vi "run vis.vi"(8 "error in (no error)":errorcluster, 11 "home path":path) -> (0 "run vis Error":errorcluster[][](array[cluster]), 2 "Panel VI names":string[](array[string]), 3 "Panel VI paths":path[](array[path]))   [LabVIEW 2016, in "main.lvlib"]
doc: "run vis.VI initializes the Control environment by opening the necessary VIs \nfor operations. \n\nBeamline section controls (main control lower panel): Both sample changers and injectors, low energy end, high energy end, transmission line, and the R30 and R45 beamlines\n\nTools (main control upper panel): monitors for terminal voltage, beam current along with BPM, foil, and other various controls.\n\nTop-level VIs (full VI's opened \"outside\" of main control): sample changer monitor/controller, vacuum readbacks, beam current monitor, cRIO monitor"
uses:
  main.lvlib
panel:
  out "Top Level open errors":errorcluster[](array[cluster])
  out "Top Level run errors":errorcluster[](array[cluster])
  out "Panel VI run errors":errorcluster[](array[cluster])
  out "Top Level paths":path[](array[path])
  out "Numeric 2":i32
  out "Numeric":i32
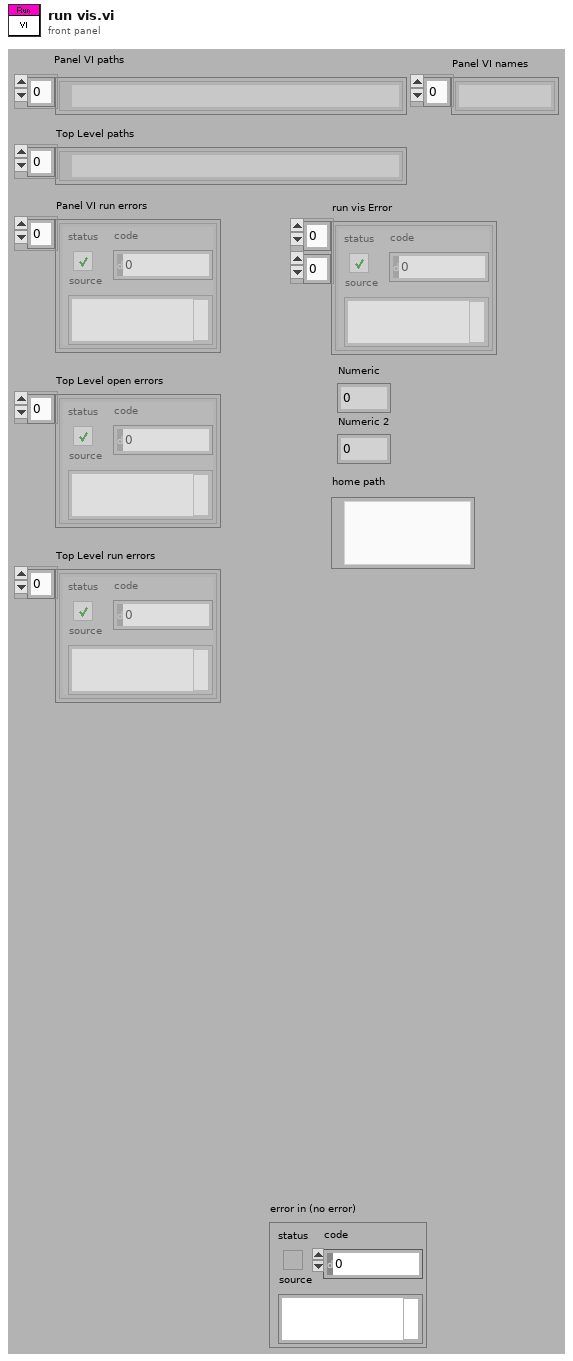
[diagram p1: front panel]
types:
  T1 = enum32{"Invalid", "Standard", "Closed", "Hidden", "Minimized", "Maximized"}
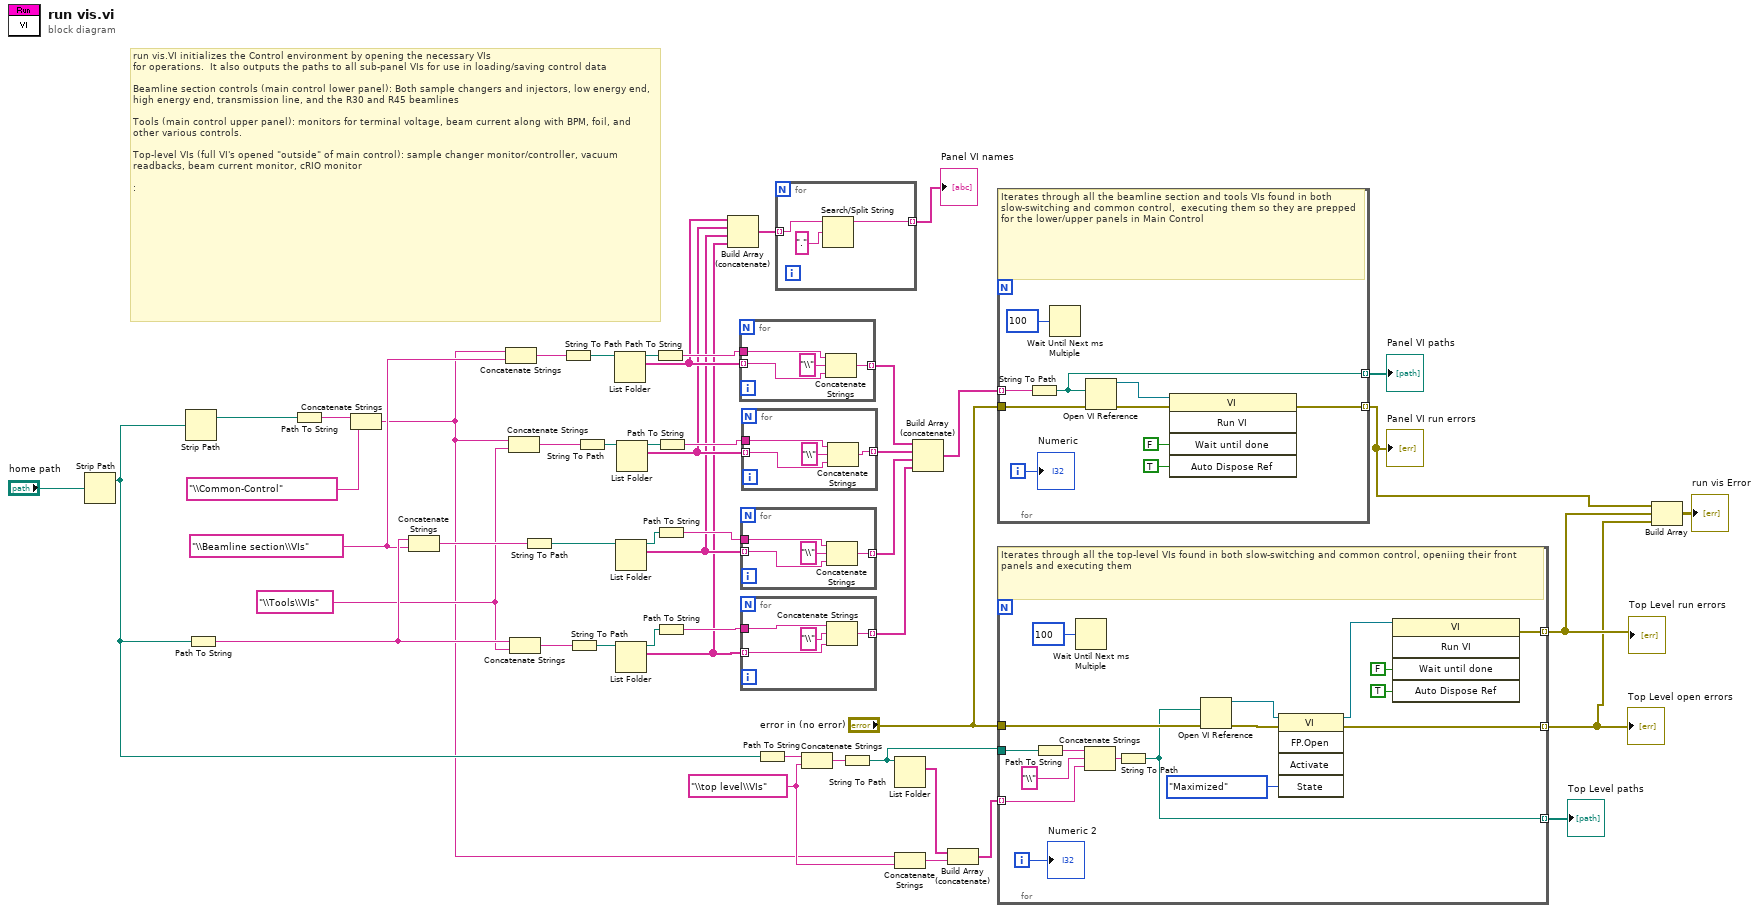
[diagram p0: block diagram]
diagram:
  w15 = "\\top level\\VIs" ("string")
  w27 = "\\Tools\\VIs" ("string")
  w28 = "\\Beamline section\\VIs" ("string")
  # "run vis.VI initializes the Control environment by opening the necessary VIs \nfor operations.  It also outputs the paths to all sub-panel VIs for use in loading/saving control data \n\nBeamline section controls (main control lower panel): Both sample changers and injectors, low energy end, high energy end, transmission line, and the R30 and R45 beamlines\n\nTools (main control upper panel): monitors for terminal voltage, beam current along with BPM, foil, and other various controls.\n\nTop-level VIs (full VI's opened \"outside\" of main control): sample changer monitor/controller, vacuum readbacks, beam current monitor, cRIO monitor\n\n:"
  n1 = Strip Path(path="home path") -> (stripped path=w31:path)  [unwired: 1 out]
  n2 = Strip Path(path=w31) -> (stripped path=w30:path)  [unwired: 1 out]
  n3 = Path To String(path=w31) -> (string=w46:string)
  n4 = Path To String(path=w30) -> (string=w29:string)
  n5 = Concatenate Strings(w29, "\\Common-Control" ("string")) -> (w14:string)
  n6 = Concatenate Strings(w46, w28) -> (w48:string)
  n7 = Concatenate Strings(w14, w28) -> (w24:string)
  n8 = Concatenate Strings(w14, w27) -> (w19:string)
  n9 = Concatenate Strings(w46, w27) -> (w45:string)
  n10 = String To Path(string=w48) -> (path=w47:path)
  n11 = String To Path(string=w24) -> (path=w23:path)
  n12 = String To Path(string=w45) -> (path=w44:path)
  n13 = String To Path(string=w19) -> (path=w20:path)
  n14 = List Folder(path=w23) -> (path out=w25:path, filenames=w6:string[])  [unwired: 3 in, 2 out]
  n15 = List Folder(path=w47) -> (path out=w34:path, filenames=w4:string[])  [unwired: 3 in, 2 out]
  n16 = List Folder(path=w44) -> (path out=w37:path, filenames=w3:string[])  [unwired: 3 in, 2 out]
  n17 = List Folder(path=w20) -> (path out=w21:path, filenames=w5:string[])  [unwired: 3 in, 2 out]
  n18 = Path To String(path=w25) -> (string=w26:string)
  n19 = Path To String(path=w34) -> (string=w35:string)
  n20 = Path To String(path=w37) -> (string=w36:string)
  n21 = Path To String(path=w21) -> (string=w22:string)
  n22 = Build Array (concatenate)(w6, w5, w4, w3) -> (w2:string[])
  n23 = for {
    tunnel: w26 -> [w54]
    tunnel: w6 -> [w52] mode=indexing
    tunnel: [w51] -> w17 mode=indexing
    n24 = Concatenate Strings(w54, "\\" ("string"), w52) -> (w51:string)
  }
  n25 = for {
    tunnel: w35 -> [w58]
    tunnel: w4 -> [w56] mode=indexing
    tunnel: [w55] -> w33 mode=indexing
    n26 = Concatenate Strings(w58, "\\" ("string"), w56) -> (w55:string)
  }
  n27 = for {
    tunnel: w36 -> [w62]
    tunnel: w3 -> [w60] mode=indexing
    tunnel: [w59] -> w32 mode=indexing
    n28 = Concatenate Strings(w62, "\\" ("string"), w60) -> (w59:string)
  }
  n29 = for {
    tunnel: w22 -> [w66]
    tunnel: w5 -> [w64] mode=indexing
    tunnel: [w63] -> w18 mode=indexing
    n30 = Concatenate Strings(w66, "\\" ("string"), w64) -> (w63:string)
  }
  n31 = Path To String(path=w31) -> (string=w42:string)
  n32 = for {
    tunnel: w2 -> [w69] mode=indexing
    tunnel: [w67] -> w1 mode=indexing
    n33 = Search/Split String(string=w69, search string/char (-)=".") -> (substring before match=w67:string)  [unwired: 1 in, 2 out]
  }
  "Panel VI names" <- w1
  n34 = Concatenate Strings(w42, w15) -> (w41:string)
  n35 = String To Path(string=w41) -> (path=w40:path)
  n36 = List Folder(path=w40) -> (filenames=w13:string[])  [unwired: 3 in, 3 out]
  n37 = Concatenate Strings(w14, w15) -> (w11:string)
  n38 = Build Array (concatenate)(w17, w18, w33, w32) -> (w43:string[])
  n39 = Build Array (concatenate)(w13, w11) -> (w12:string[])
  n40 = for {
    tunnel: "error in (no error)" -> [w74]
    tunnel: w43 -> [w71] mode=indexing
    tunnel: [w72] -> w39 mode=indexing
    tunnel: [w70] -> w10 mode=indexing
    i -> [w73]
    # "Iterates through all the beamline section and tools VIs found in both slow-switching and common control,  executing them so they are prepped for the lower/upper panels in Main Control"
    n41 = String To Path(string=w71) -> (path=w72:path)
    n42 = Wait Until Next ms Multiple(millisecond multiple=u32 100) -> ()  [unwired: 1 out]
    n43 = Open VI Reference(vi path=w72, error in (no error)=w74) -> (vi reference=w79:refnum<vi>, error out=w75:errorcluster)  [unwired: 1 in, 3 out]
    n44 = invoke class="VI" method="Run VI"(reference=w79, error in=w75, "Wait until done"=FALSE ("Wait Until Done"), "Auto Dispose Ref"=TRUE ("Auto Dispose Reference")) -> (error out=w70:errorcluster)  [unwired: 1 in, 4 out]
    "Numeric" <- w73
  }
  "Panel VI paths" <- w39
  "Panel VI run errors" <- w10
  n45 = for {
    tunnel: "error in (no error)" -> [w93]
    tunnel: w12 -> [w83] mode=indexing
    tunnel: w40 -> [w86]
    tunnel: [w84] -> w38 mode=indexing
    tunnel: [w81] -> w9 mode=indexing
    tunnel: [w80] -> w8 mode=indexing
    i -> [w85]
    # "Iterates through all the top-level VIs found in both slow-switching and common control, openiing their front panels and executing them"
    n46 = Path To String(path=w86) -> (string=w87:string)
    n47 = Wait Until Next ms Multiple(millisecond multiple=u32 100) -> ()  [unwired: 1 out]
    n48 = Concatenate Strings(w87, "\\" ("string"), w83) -> (w88:string)
    n49 = String To Path(string=w88) -> (path=w84:path)
    n50 = Open VI Reference(vi path=w84, error in (no error)=w93) -> (vi reference=w91:refnum<vi>, error out=w90:errorcluster)  [unwired: 1 in, 3 out]
    n51 = invoke class="VI" method="FP.Open"(reference=w91, error in=w90, "State"=T1."Maximized") -> (reference out=w89:refnum<vi>, error out=w80:errorcluster)  [unwired: 2 in, 3 out]
    n52 = invoke class="VI" method="Run VI"(reference=w89, "Wait until done"=FALSE ("Wait Until Done"), "Auto Dispose Ref"=TRUE ("Auto Dispose Reference")) -> (error out=w81:errorcluster)  [unwired: 2 in, 4 out]
    "Numeric 2" <- w85
  }
  "Top Level paths" <- w38
  "Top Level run errors" <- w9
  "Top Level open errors" <- w8
  n53 = Build Array(w10, w9, w8) -> (→"run vis Error":errorcluster[][])
